vi "Get Asic Type Name.vi"(8 "error in (no error)":errorcluster caption="错误输入（无错误）", 11 "asicType":i32) -> (0 "error out":errorcluster caption="错误输出", 3 "function return":string)   [LabVIEW 2018]
doc: "extern char * __stdcall APSxGetAsicTypeName (int asicType);"
uses:
  APSx.dll/APSx.dll
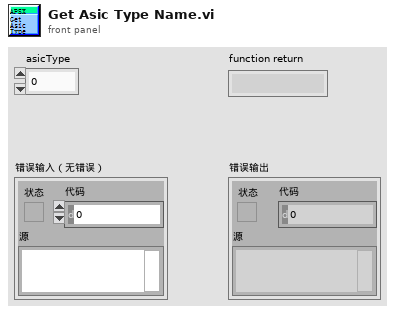
[diagram p1: front panel]
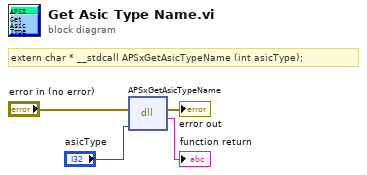
[diagram p0: block diagram]
diagram:
  # "extern char * __stdcall APSxGetAsicTypeName (int asicType);"
  n1 = dll-call lib="PTH2[abs D项目Feng恒隆项目Labview传感器对中台SourcesAPSx.dllAPSx.*" fn="APSxGetAsicTypeName"(error in="error in (no error)", "asicType"="asicType") -> (error out=→"error out":errorcluster, →"function return":string)  [unwired: 3 in, 1 out]
